vi "TestRFGVPersonnel.vi"(10 "Rooms":i32=101) -> ()   [LabVIEW 2015]
uses:
  TypeDef/RoomsActionEnum.ctl
panel:
  out "Remove":bool
  out "Add":bool
  out "Add Personnel 2":string
  out "Read Personnel 3":string
  out "Remove Personnel":string
  out "Add Personnel 1":string
  out "Read Personnel 1":string
  out "Read Personnel 2":string
  out "error out":errorcluster
  out "Pass":bool
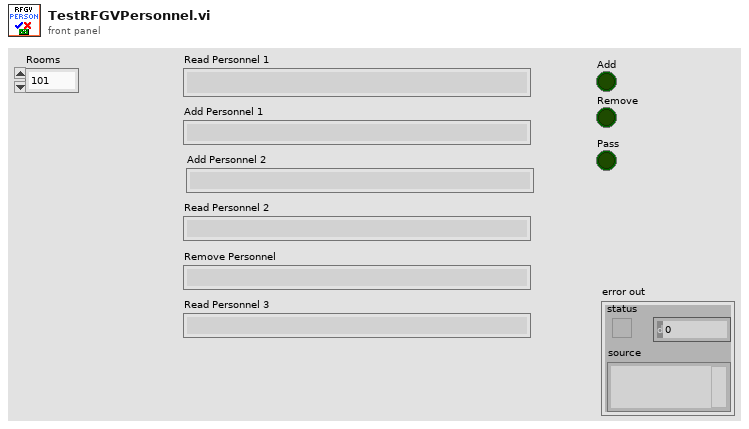
[diagram p1: front panel]
types:
  T1 = typedef "RoomsActionEnum.ctl" = enum16{"Init", "Add Room", "Remove Room", "Read Room", "Read Flag", "Read Flag State", "Write Flag State", "Read Flag Color", "Write Flag Color", "Read Bed Vacant", "Write Bed Vacant", "Read Personnel", "Add Personnel", "Remove Personnel", "Read Requests", "Add Request", "Remove Request", "Read Beacon ID", "Write Beacon ID", "Write Bed URL", "Read Bed URL", "Read Rooms Numbers", "Write Flag"}
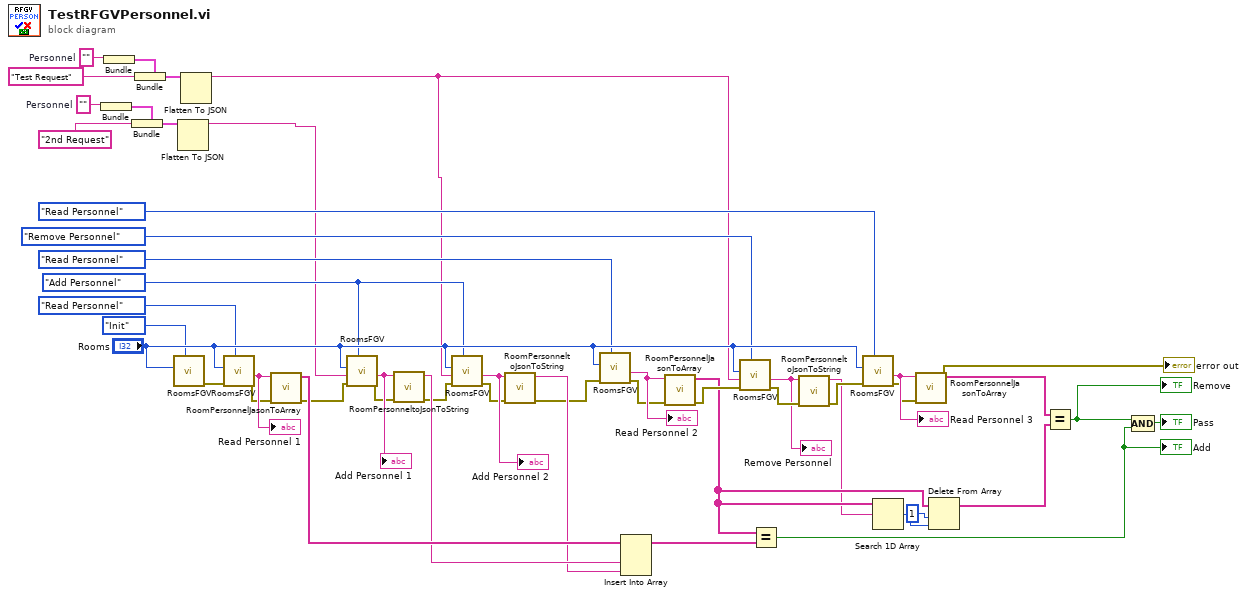
[diagram p0: block diagram]
diagram:
  w6 = RoomsActionEnum."Add Personnel" ("Actions")
  w42 = ""  # Personnel
  w49 = ""  # Personnel
  n1 = Bundle("Personnel"=w42) -> (w43:cluster{"Personnel":string})  [unwired: 1 in]
  n2 = Bundle("Personnel"=w49) -> (w48:cluster{"Personnel":string})  [unwired: 1 in]
  n3 = Bundle(cluster=w43, "Personnel"="2nd Request" ("Request 2")) -> (w44:cluster{"Personnel":string})
  n4 = Bundle(cluster=w48, "Personnel"="Test Request" ("Request")) -> (w47:cluster{"Personnel":string})
  n5 = call "RoomsFGV.vi"("Actions"=RoomsActionEnum."Init", "Room"="Rooms") -> ("error out"=w41:errorcluster)  [unwired: 8 in, 1 out]
  n6 = Flatten To JSON(anything=w44) -> (JSON string=w2:string)  [unwired: 2 in, 1 out]
  n7 = Flatten To JSON(anything=w47) -> (JSON string=w1:string)  [unwired: 2 in, 1 out]
  n8 = call "RoomsFGV.vi"("Actions"=RoomsActionEnum."Read Personnel", "error in (no error)"=w41, "Room"="Rooms") -> ("error out"=w30:errorcluster, "Data Out"=w36:string)  [unwired: 7 in]
  "Read Personnel 1" <- w36
  n9 = call "RoomPersonnelJasonToArray.vi"("error in (no error)"=w30, "Data Out"=w36) -> ("error out"=w29:errorcluster, "REQs"=w35:string[])  [unwired: 8 in]
  n10 = call "RoomsFGV.vi"("Actions"=w6, "error in (no error)"=w29, "Data In"=w2, "Room"="Rooms") -> ("error out"=w28:errorcluster, "Data Out"=w38:string)  [unwired: 6 in]
  "Add Personnel 1" <- w38
  n11 = call "RoomPersonneltoJsonToString.vi"("error in (no error)"=w28, "Data Out"=w38) -> ("error out"=w27:errorcluster, "Request"=w34:string)  [unwired: 8 in]
  n12 = call "RoomsFGV.vi"("Actions"=w6, "error in (no error)"=w27, "Data In"=w1, "Room"="Rooms") -> ("error out"=w26:errorcluster, "Data Out"=w37:string)  [unwired: 6 in]
  "Add Personnel 2" <- w37
  n13 = call "RoomPersonneltoJsonToString.vi"("error in (no error)"=w26, "Data Out"=w37) -> ("error out"=w25:errorcluster, "Request"=w33:string)  [unwired: 8 in]
  n14 = call "RoomsFGV.vi"("Actions"=RoomsActionEnum."Read Personnel", "error in (no error)"=w25, "Room"="Rooms") -> ("error out"=w24:errorcluster, "Data Out"=w32:string)  [unwired: 7 in]
  "Read Personnel 2" <- w32
  n15 = Insert Into Array(array=w35, new element #1=w34, new element #2=w33) -> (w31:string[])  [unwired: 1 in]
  n16 = call "RoomPersonnelJasonToArray.vi"("error in (no error)"=w24, "Data Out"=w32) -> ("error out"=w23:errorcluster, "REQs"=w17:string[])  [unwired: 8 in]
  n17 = call "RoomsFGV.vi"("Actions"=RoomsActionEnum."Remove Personnel", "error in (no error)"=w23, "Data In"=w1, "Room"="Rooms") -> ("error out"=w22:errorcluster, "Data Out"=w20:string)  [unwired: 6 in]
  "Remove Personnel" <- w20
  n18 = Equal?(x=w17, y=w31) -> (x = y?=w39:bool)
  "Add" <- w39
  n19 = call "RoomPersonneltoJsonToString.vi"("error in (no error)"=w22, "Data Out"=w20) -> ("error out"=w21:errorcluster, "Request"=w16:string)  [unwired: 8 in]
  n20 = call "RoomsFGV.vi"("Actions"=RoomsActionEnum."Read Personnel", "error in (no error)"=w21, "Room"="Rooms") -> ("error out"=w14:errorcluster, "Data Out"=w15:string)  [unwired: 7 in]
  "Read Personnel 3" <- w15
  n21 = Search 1D Array(1D array=w17, element=w16) -> (index of element=w19:i32)  [unwired: 1 in]
  n22 = call "RoomPersonnelJasonToArray.vi"("error in (no error)"=w14, "Data Out"=w15) -> ("error out"=→"error out":errorcluster, "REQs"=w12:string[])  [unwired: 8 in]
  n23 = Delete From Array(array=w17, length=1, index=w19) -> (array with subset deleted=w11:string[])  [unwired: 1 out]
  n24 = Equal?(x=w12, y=w11) -> (x = y?=w40:bool)
  "Remove" <- w40
  n25 = Compound Arithmetic op=AND(w40, w39) -> (→"Pass":bool)
